vi "Read Serial Output Channel Status.vi"(0 "fpga interface in":refnum<k20>, 11 "error in (no error)":errorcluster) -> (4 "fpga interface out":refnum<k20>, 6 "serial output channel status":T1(array[cluster]), 15 "error out":errorcluster)   [LabVIEW 2023, in "GettingStarted_Gen_148X_Host.lvlib"]
uses:
  GettingStarted_Gen_148X_Host.lvlib
  Types/148x_Gen_FPGA_Reference.ctl
  <vilib>/Utility/error.llb/Error Cluster From Error Code.vi
  <vilib>/rvi/errors/niLvFpgaAdjustHostInterfaceError.vi
  <vilib>/rvi/interface/nirviReadWriteControl/nirviReadWriteControl.xnode
  NiFpgaLv.dll
  <vilib>/rvi/interface/Simulation/niFpgaSimulationCallBeginRW.vi
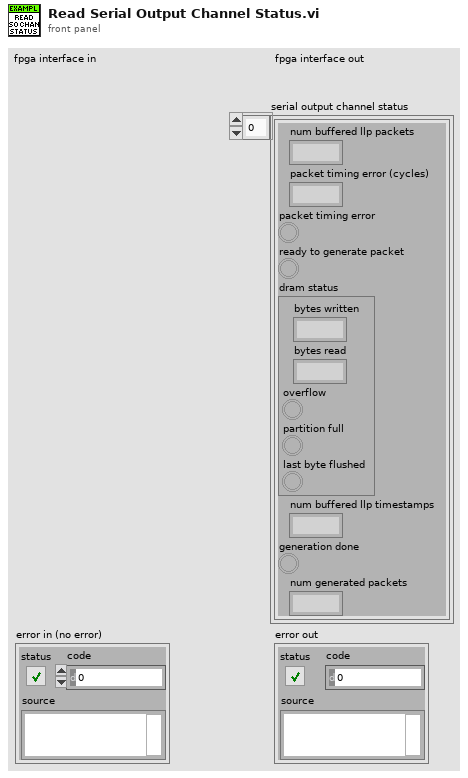
[diagram p1: front panel]
types:
  T1 = cluster{"num buffered llp packets":fxp<+,14,14>, "packet timing error (cycles)":u64, "packet timing error":bool, "ready to generate packet":bool, "dram status":cluster{"bytes written":u64, "bytes read":u64, "overflow":bool, "partition full":bool, "last byte flushed":bool}, "num buffered llp timestamps":u32, "generation done":bool, "num generated packets":u64}[]
  T2 = typedef "GettingStarted_Gen_148X_Host.lvlib/148x_Gen_FPGA_Reference.ctl" = refnum<k20>
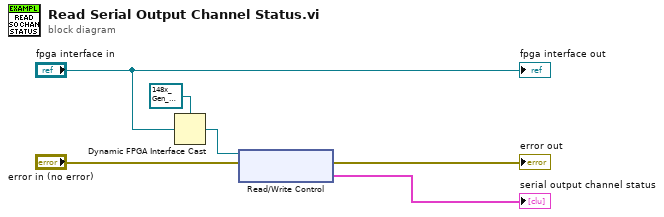
[diagram p0: block diagram]
diagram:
  n1 = Dynamic FPGA Interface Cast(Session In=T2 refnum ("FPGA VI Reference Out"), Type="fpga interface in") -> (Session Out=w6:T2)
  n2 = xnode "Read/Write Control"("FPGA VI Reference In"=w6, "error in"="error in (no error)") -> ("error out"=→"error out":errorcluster, "channel status"=→"serial output channel status":T1)  [unwired: 1 out]
  "fpga interface out" <- "fpga interface in"
